vi "呈现图片.vi"(8 "error in (no error)":errorcluster caption="错误输入（无错误）", 11 "集合 输入":refnum<class "集合.lvclass"> caption="DNL_LabVIEW Object in") -> (0 "error out":errorcluster caption="错误输出", 2 "Picture":picture caption="图片", 3 "集合 输出":refnum<class "集合.lvclass"> caption="DNL_LabVIEW Object out")   [LabVIEW 2011, in "集合.lvclass"]
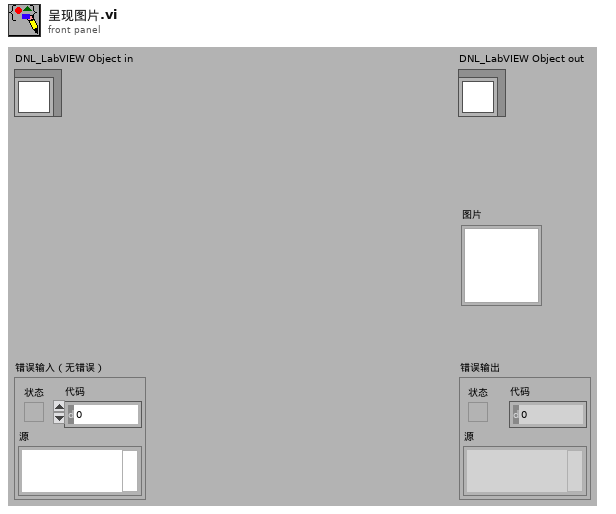
[diagram p1: front panel]
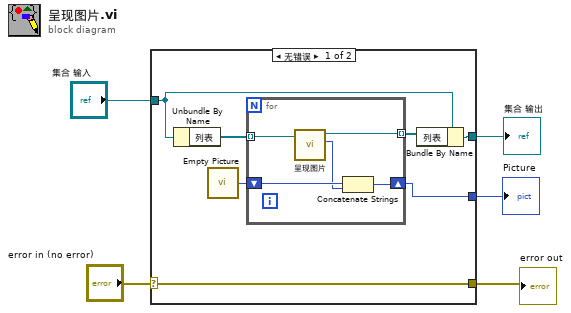
[diagram p0: block diagram]
diagram:
  n1 = case shown="无错误" "error in (no error)" {
    selector: "error in (no error)" -> [w12 w18]
    tunnel: [w12 w18] -> w4
    tunnel: "集合 输入" -> [w9 w19]
    tunnel: [w8 w19] -> w2
    tunnel: [w6 _] -> w1
    frame No Error {
      n2 = Unbundle By Name(w9) -> ("列表"=w11:refnum<class "图形.lvclass">[])
      n3 = call "Empty Picture"() -> ("empty picture"=w7:picture)
      n4 = for {
        tunnel: w11 -> [w17] mode=indexing
        tunnel: [w16] -> w10 mode=indexing
        shift-right: [w14] -> w6
        shift-left: w7 -> [w15]
        n5 = call-dynamic "呈现图片.vi"("图形 输入"=w17) -> ("Picture"=w13:picture, "图形 输出"=w16:refnum<class "图形.lvclass">)  [unwired: 8 in, 1 out]
        n6 = Concatenate Strings(w15, w13) -> (w14:picture)
      }
      n7 = Bundle By Name(cluster=w9, "列表"=w10) -> (w8:refnum<class "集合.lvclass">)
    }
    frame Error {
    }
  }
  "error out" <- w4
  "集合 输出" <- w2
  "Picture" <- w1
